vi "XY Graph Get Selected Plot.vi"(8 "error in (no error)":errorcluster, 11 "Selected Plot Info":T2) -> (0 "error out":errorcluster, 1 "Plot Name":string, 2 "Plot Index":i32, 3 "Plot":T1, 4 "Plot Index in (dup)":i32, 5 "Graph Name":string)   [LabVIEW 2021, in "XY Graph Add-Ons.lvlib"]
uses:
  XY Graph Add-Ons.lvlib
  XY Graph Selected Plot Info.ctl
  XY Graph Refnum.ctl
  <vilib>/Utility/miscctls.llb/LVPoint32TypeDef.ctl
  XY Plot Data.ctl
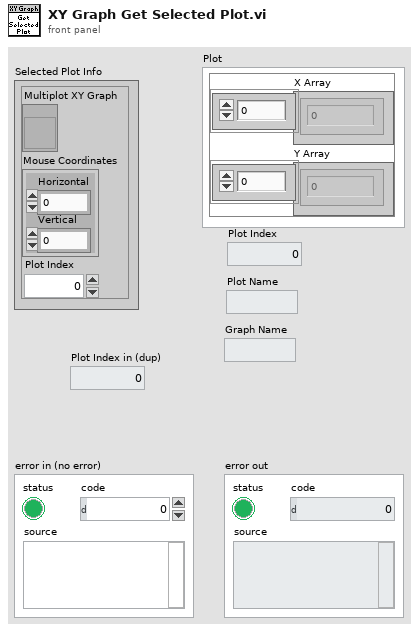
[diagram p1: front panel]
types:
  T1 = typedef "XY Graph Add-Ons.lvlib/XY Plot Data.ctl" = cluster{"X Array":dbl[], "Y Array":dbl[]}
  T2 = typedef "XY Graph Add-Ons.lvlib/XY Graph Selected Plot Info.ctl" = cluster{"Multiplot XY Graph":T3, "Mouse Coordinates":T4, "Plot Index":i32}
  T3 = typedef "XY Graph Add-Ons.lvlib/XY Graph Refnum.ctl" = refnum<vi>
  T4 = typedef "LVPoint32TypeDef.ctl" = cluster{"Horizontal":i32, "Vertical":i32}
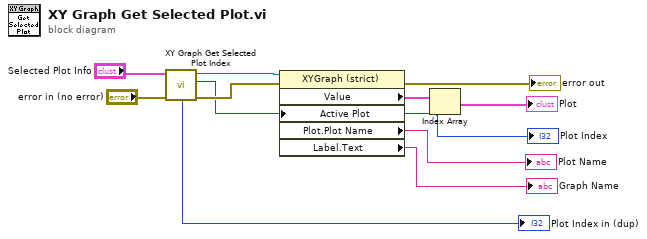
[diagram p0: block diagram]
diagram:
  n1 = call "XY Graph Get Selected Plot Index.vi"("error in (no error)"="error in (no error)", "Selected Plot Info"="Selected Plot Info") -> ("error out"=w4:errorcluster, "Plot at Coordinates"=w2:i32, "XYGraph out"=w3:T3, "Plot Index in (dup)"=→"Plot Index in (dup)":i32)  [unwired: 6 in]
  "Plot Index" <- w2
  n2 = property class="XYGraph (strict)"(reference=w3, error in=w4, "Active Plot"=w2) -> (error out=→"error out":errorcluster, "Value"=w5:cluster{"X Array":dbl[], "Y Array":dbl[]}[], "Plot.Plot Name"=→"Plot Name":string, "Label.Text"=→"Graph Name":string)  [unwired: 1 out]
  n3 = Index Array(array=w5, index=w2) -> (element=→"Plot":cluster{"X Array":dbl[], "Y Array":dbl[]})
